vi "Color to RGBA.vi"(0 "Color Box":u32(colorbox)) -> (1 "R":u8, 2 "G":u8, 3 "B":u8, 4 "A":u8)   [LabVIEW 2023, in "Glyph Drawer.lvlib"]
uses:
  Glyph Drawer.lvlib
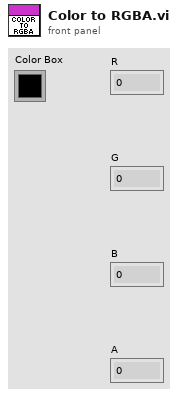
[diagram p1: front panel]
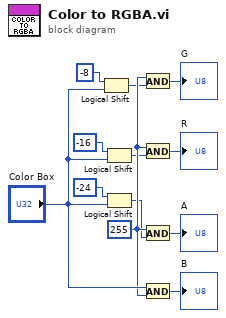
[diagram p0: block diagram]
diagram:
  w7 = u32 255
  n1 = Logical Shift(y=i16 -8, x="Color Box") -> (x << y=w4:u32)
  n2 = Logical Shift(y=i16 -16, x="Color Box") -> (x << y=w5:u32)
  n3 = Logical Shift(y=i16 -24, x="Color Box") -> (x << y=w6:u32)
  n4 = And(x=w7, y=w4) -> (x .and. y?=→"G":u32)
  n5 = And(x=w7, y=w5) -> (x .and. y?=→"R":u32)
  n6 = And(x=w7, y=w6) -> (x .and. y?=→"A":u32)
  n7 = And(x="Color Box", y=w7) -> (x .and. y?=→"B":u32)
